vi "fgv_module_error.vi"(7 "cmd":T1=enum."TIM571 error in", 9 "PwrPak7 error in":errorcluster, 10 "tim571 error in":errorcluster, 11 "vlp16 error in":errorcluster) -> (1 "PwrPak7 error out":errorcluster caption="PwrPak7 error in", 2 "tim571 error out":errorcluster caption="tim571 error in", 3 "vlp16 error out":errorcluster caption="vlp16 error in")   [LabVIEW 2019]
uses:
  Ctrl/error_modules.ctl
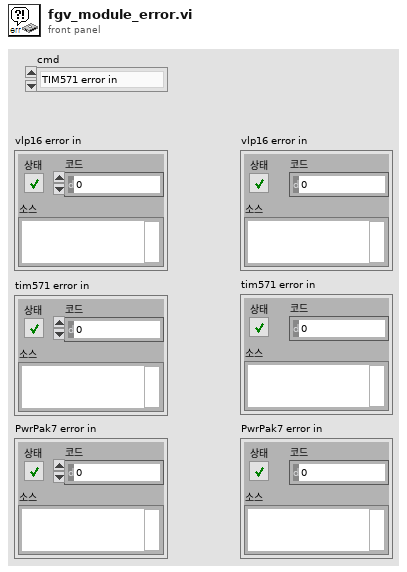
[diagram p1: front panel]
types:
  T1 = typedef "error_modules.ctl" = enum16{"init", "read", "TIM571 error in", "VLP16 error in", "PwrPak7 error in"}
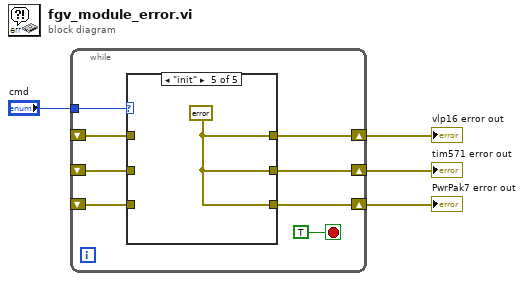
[diagram p0: block diagram]
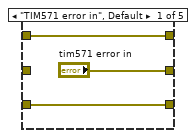
[diagram p2: hidden frame]
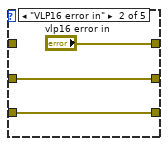
[diagram p3: hidden frame]
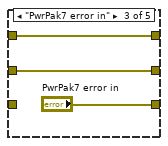
[diagram p4: hidden frame]
diagram:
  n1 = while {
    tunnel: "cmd" -> [w11]
    shift-right: [w10] -> w3
    shift-left: _ -> [w5]
    shift-right: [w9] -> w2
    shift-left: _ -> [w8]
    shift-right: [w7] -> w1
    shift-left: _ -> [w6]
    stop <- TRUE stop-if-true
    n2 = case shown="\"init\"" w11 {
      tunnel: [w15 "vlp16 error in" w19 w24 w25] -> w10
      tunnel: ["tim571 error in" w17 w20 w23 w25] -> w9
      tunnel: w8 -> [_ w17 w20 w23 _]
      tunnel: [w13 w16 "PwrPak7 error in" w22 w25] -> w7
      tunnel: w6 -> [w13 w16 _ w22 _]
      tunnel: w5 -> [w15 _ w19 w24 _]
      frame "TIM571 error in", Default {
      }
      frame "VLP16 error in" {
      }
      frame "PwrPak7 error in" {
      }
      frame "read" {
      }
      frame "init" {
        w25 = errorcluster {"status"=FALSE, "code"=0, "source"=""} ("vlp16 error in")
      }
    }
  }
  "vlp16 error out" <- w3
  "tim571 error out" <- w2
  "PwrPak7 error out" <- w1
